vi "OpenAnotherOne.vi"(8 "error in (no error)":errorcluster, 9 "Reverse Solenoid Channel":T1=enum."Solenoid 1", 10 "Forward Solenoid Channel":T1, 11 "Pneumatics Control Module (0)":u8) -> (0 "error out":errorcluster, 3 "SolenoidDevRef":T2={"DevStatus"={"status"=FALSE, "code"=0, "source"=""}, "Pneumatics Control Module"=0, "Forward Solenoid Channel"=enum."Invalid", "Reverse Solenoid Channel"=enum."Invalid"})   [LabVIEW 2015]
uses:
  <vilib>/Rock Robotics/WPI/Solenoid/WPI_SolenoidDevRef.ctl
  <vilib>/Rock Robotics/WPI/Solenoid/WPI_SolenoidChannel.ctl
  <vilib>/Rock Robotics/WPI/Solenoid/WPI_SolenoidCacheOp.ctl
  <vilib>/Rock Robotics/SystemInterfaces/NetworkCommunication/NetComm_UsageReport_ResourceType.ctl
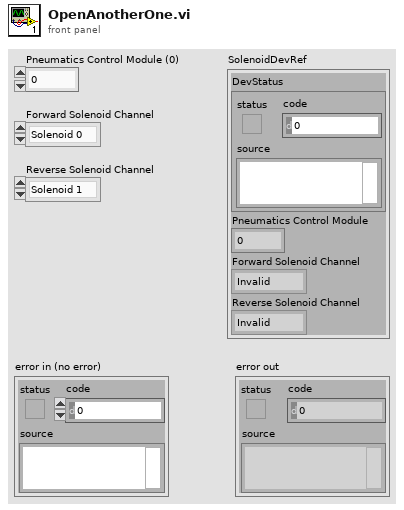
[diagram p1: front panel]
types:
  T1 = typedef "WPI_SolenoidChannel.ctl" = enum8{"Solenoid 0", "Solenoid 1", "Solenoid 2", "Solenoid 3", "Solenoid 4", "Solenoid 5", "Solenoid 6", "Solenoid 7", "Invalid"}
  T2 = typedef "WPI_SolenoidDevRef.ctl" = cluster{"DevStatus":errorcluster, "Pneumatics Control Module":u8, "Forward Solenoid Channel":T1, "Reverse Solenoid Channel":T1}
  T3 = typedef "WPI_SolenoidCacheOp.ctl" = enum16{"Acquire", "Release", "Status"}
  T4 = typedef "NetComm_UsageReport_ResourceType.ctl" = enum8{"Controller", "Module", "Language", "CANPlugin", "Accelerometer", "ADXL345", "AnalogChannel", "AnalogTrigger", "AnalogTriggerOutput", "CANJaguar", "Compressor", "Counter", "Dashboard", "DigitalInput", "DigitalOutput", "DriverStationCIO", "DriverStationEIO", "DriverStationLCD", "Encoder", "GearTooth", "Gyro", "I2C", "Framework", "Jaguar", "Joystick", "Kinect", "KinectStick", "PIDController", "Preferences", "PWM", "Relay", "RobotDrive", "SerialPort", "Servo", "Solenoid", "SPI", "Task", "Ultrasonic", "Victor", "Button", "Command", "AxisCamera", "PCVideoServer", "SmartDashboard", "Talon", "HiTechnicColorSensor", "HiTechnicAccel", "HiTechnicCompass", "SRF08", "AnalogOutput", "Victor SP", "Talon SRX", "CAN Talon SRX", "ADXL362 Accel", "ADXRS450 Gyro", "Rev SPARK", "Mindsensors SD540", "Digital Filter"}
  T5 = typedef "WPI_CompressorDevRef.ctl" = cluster{"DevStatus":errorcluster, "Pneumatics Control Module":u8}
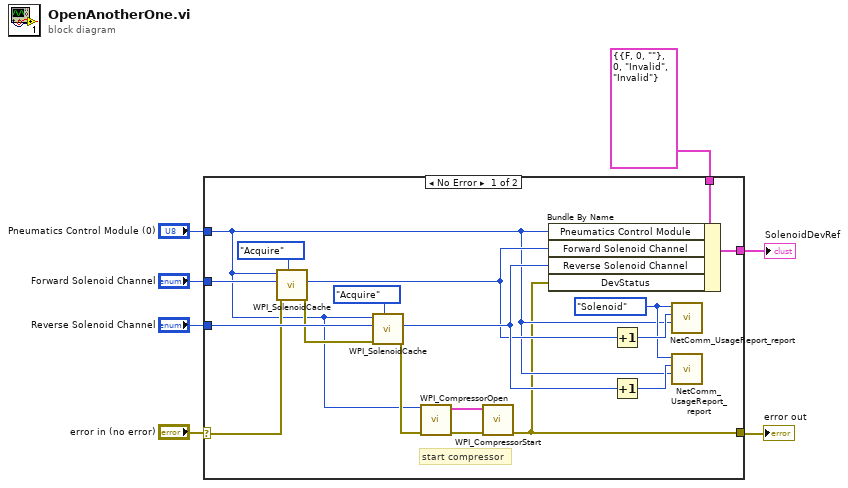
[diagram p0: block diagram]
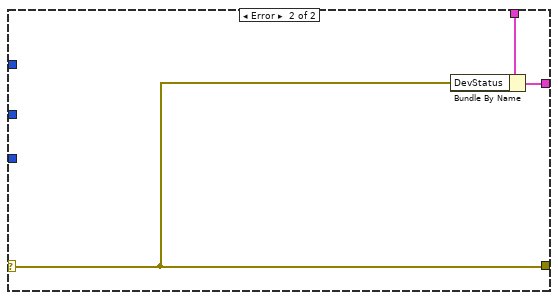
[diagram p2: hidden frame]
diagram:
  n1 = case shown="No Error" "error in (no error)" {
    selector: "error in (no error)" -> [w14 w26]
    tunnel: [w8 w26] -> w6
    tunnel: [w24 w28] -> w4
    tunnel: "Forward Solenoid Channel" -> [w22 _]
    tunnel: "Pneumatics Control Module (0)" -> [w9 _]
    tunnel: T2 {"DevStatus"={"status"=FALSE, "code"=0, "source"=""}, "Pneumatics Control Module"=0, "Forward Solenoid Channel"=enum."Invalid", "Reverse Solenoid Channel"=enum."Invalid"} ("SolenoidDevRef") -> [w25 w27]
    tunnel: "Reverse Solenoid Channel" -> [w20 _]
    frame No Error {
      w17 = NetComm_UsageReport_ResourceType."Solenoid" ("Resource Type")
      # "start compressor"
      n2 = call <vilib>:"WPI_SolenoidCache.vi"("AllocatedSolenoidOp"=WPI_SolenoidCacheOp."Acquire", "error in (no error)"=w14, "SolenoidChannel"=w22, "Pneumatics Control Module"=w9) -> ("error out"=w13:errorcluster, "AllocatedSolenoidChannel"=w15:T1)  [unwired: 1 in, 5 out]
      n3 = call <vilib>:"WPI_SolenoidCache.vi"("AllocatedSolenoidOp"=WPI_SolenoidCacheOp."Acquire", "error in (no error)"=w13, "SolenoidChannel"=w20, "Pneumatics Control Module"=w9) -> ("error out"=w10:errorcluster, "AllocatedSolenoidChannel"=w16:T1)  [unwired: 1 in, 5 out]
      n4 = call <vilib>:"WPI_CompressorOpen.vi"("Pneumatics Control Module (0)"=w9, "error in (no error)"=w10) -> ("CompressorDevRef"=w12:T5, "error out"=w11:errorcluster)  [unwired: 12 in]
      n5 = call <vilib>:"WPI_CompressorStart.vi"("error in (no error)"=w11, "CompressorDevRef"=w12) -> ("error out"=w8:errorcluster)  [unwired: 8 in, 1 out]
      n6 = Bundle By Name(cluster=w25, "Pneumatics Control Module"=w9, "Forward Solenoid Channel"=w15, "Reverse Solenoid Channel"=w16, "DevStatus"=w8) -> (w24:T2)
      n7 = Increment(x=w15) -> (x+1=w19:T1)
      n8 = Increment(x=w16) -> (x+1=w18:T1)
      n9 = call <vilib>:"NetComm_UsageReport_report.vi"("Context"=w9, "Instance Number"=w19, "Resource Type"=w17) -> ()  [unwired: 9 in]
      n10 = call <vilib>:"NetComm_UsageReport_report.vi"("Context"=w9, "Instance Number"=w18, "Resource Type"=w17) -> ()  [unwired: 9 in]
    }
    frame Error {
      n11 = Bundle By Name(cluster=w27, "DevStatus"=w26) -> (w28:T2)
    }
  }
  "SolenoidDevRef" <- w4
  "error out" <- w6
